vi "convert_float_array_to_U8_Picture.vi"(7 "Pict Refnum":refnum<vi>, 8 "error in (no error)":errorcluster, 9 "planeToDisplayFeatures":enum16{"XY", "XZ", "YZ"}(ring), 10 "FEATURES (PIX)":sgl[][](array[numeric]), 11 "HOLO":sgl[][](array[numeric])) -> (0 "error out":errorcluster, 3 "new picture":picture)   [LabVIEW 2023, in "holoPyTracks.lvlib"]
uses:
  holoPyTracks.lvlib
panel:
  in  "LOG?":bool=TRUE
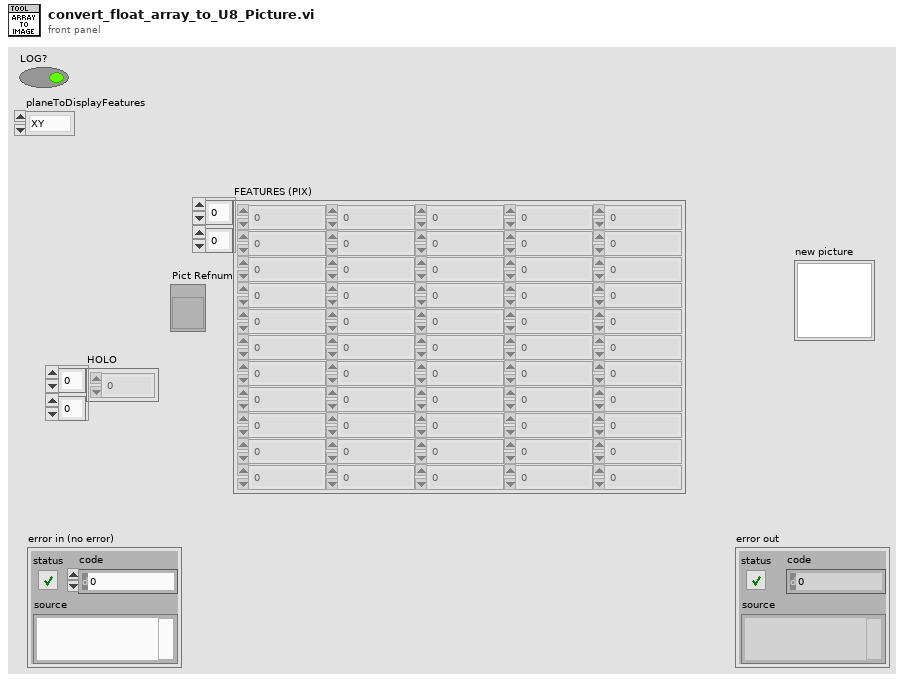
[diagram p1: front panel]
types:
  T1 = typedef "LVBoundsTypeDef.ctl" = cluster{"Width":u32, "Height":u32}
  T2 = typedef "imagedata.ctl" = cluster{"image type":i32, "image depth":i32, "image":u8[], "mask":u8[], "colors":u32[], "Rectangle":cluster{"left":i16, "top":i16, "right":i16, "bottom":i16}}
  T3 = cluster{"Width":u16, "Style":enum32{"Solid", "Dash", "Dot", "DashDot", "DashDotDot"}}
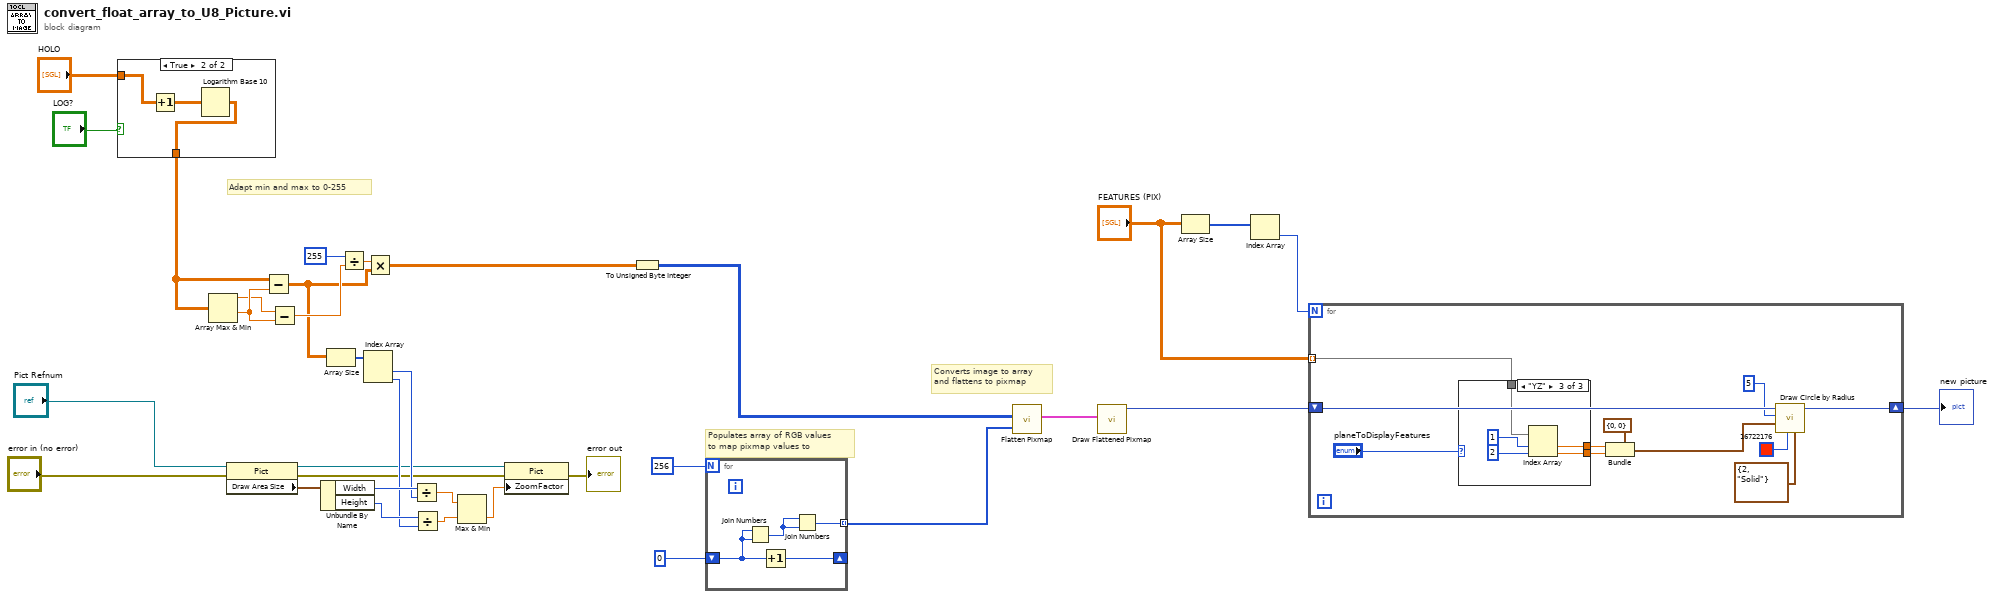
[diagram p0: block diagram]
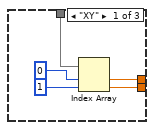
[diagram p3: hidden frame]
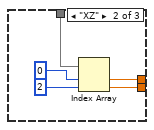
[diagram p4: hidden frame]
diagram:
  # "Adapt min and max to 0-255"
  # "Converts image to array\nand flattens to pixmap"
  # "Populates array of RGB values\nto map pixmap values to"
  n1 = case shown="True" "LOG?" {
    tunnel: "HOLO" -> [w35 w37]
    tunnel: [w35 w36] -> w2
    frame False {
    }
    frame True {
      n2 = Increment(x=w37) -> (x+1=w38:sgl[][])
      n3 = Logarithm Base 10(1:w38) -> (0:w36:sgl[][])
    }
  }
  n4 = Array Max & Min(array=w2) -> (max value=w26:sgl, min value=w27:sgl)  [unwired: 2 out]
  n5 = property on="Property Node" class="Pict"(reference="Pict Refnum", error in="error in (no error)") -> (reference out=w6:refnum<vi>, error out=w7:errorcluster, "Draw Area Size"=w24:T1)
  n6 = Subtract(x=w2, y=w27) -> (x-y=w15:sgl[][])
  n7 = Subtract(x=w26, y=w27) -> (x-y=w28:sgl)
  n8 = Unbundle By Name(w24) -> ("Width"=w23:u32, "Height"=w22:u32)
  n9 = Array Size(array=w15) -> (size(s)=w21:i32[])
  n10 = Divide(x=255, y=w28) -> (x/y=w29:sgl)
  n11 = Index Array(array=w21) -> (element #1=w20:i32, element #2=w19:i32)  [unwired: 2 in]
  n12 = Multiply(x=w29, y=w15) -> (x*y=w4:sgl[][])
  n13 = Divide(x=w23, y=w20) -> (x/y=w17:dbl)
  n14 = Divide(x=w22, y=w19) -> (x/y=w18:dbl)
  n15 = Max & Min(x=w17, y=w18) -> (min(x,y)=w16:dbl)  [unwired: 1 out]
  n16 = property on="Property Node" class="Pict"(reference=w6, error in=w7, "ZoomFactor"=w16) -> (error out=→"error out":errorcluster)  [unwired: 1 out]
  n17 = To Unsigned Byte Integer(number=w4) -> (unsigned 8bit integer=w34:u8[][])
  n18 = for {
    N: 256 -> [_]
    tunnel: [w42] -> w31 mode=indexing
    shift-right: [w41] -> _
    shift-left: u8 0 -> [w39]
    n19 = Join Numbers(hi=w39, lo=w39) -> ((hi.lo)=w40:u16)
    n20 = Increment(x=w39) -> (x+1=w41:u8)
    n21 = Join Numbers(hi=w40, lo=w40) -> ((hi.lo)=w42:u32)
  }
  n22 = call <vilib>:"Flatten Pixmap.vi"("colors"=w31, "8-bit pixmap"=w34) -> ("image data"=w30:T2)  [unwired: 9 in]
  n23 = call <vilib>:"Draw Flattened Pixmap.vi"("image data"=w30) -> ("new picture"=w14:picture)  [unwired: 8 in]
  n24 = Array Size(array="FEATURES (PIX)") -> (size(s)=w12:i32[])
  n25 = Index Array(array=w12) -> (element=w11:i32)  [unwired: 1 in]
  n26 = for {
    N: w11 -> [_]
    shift-right: [w52] -> w13
    shift-left: w14 -> [w53]
    tunnel: "FEATURES (PIX)" -> [w51] mode=indexing
    n27 = case shown="\"YZ\"" "planeToDisplayFeatures" {
      tunnel: w51 -> [w58 w63 w68]
      tunnel: [w55 w60 w65] -> w50
      tunnel: [w54 w59 w64] -> w49
      frame "XY" {
        n28 = Index Array(array=w58, index #1=0 ("disabled index (col)"), index #2=1 ("index (col)")) -> (element #1=w54:sgl, element #2=w55:sgl)
      }
      frame "XZ" {
        n29 = Index Array(array=w63, index #1=0 ("disabled index (col)"), index #2=2 ("index (col)")) -> (element #1=w59:sgl, element #2=w60:sgl)
      }
      frame "YZ" {
        n30 = Index Array(array=w68, index #1=1 ("disabled index (col)"), index #2=2 ("index (col)")) -> (element #1=w64:sgl, element #2=w65:sgl)
      }
    }
    n31 = Bundle(cluster=cluster{"horizontal":i16, "vertical":i16} {"horizontal"=0, "vertical"=0} ("pixel center"), "horizontal"=w49, "vertical"=w50) -> (w47:cluster{"horizontal":i16, "vertical":i16})
    n32 = call <vilib>:"Draw Circle by Radius.vi"("pen"=T3 {"Width"=2, "Style"=enum."Solid"}, "color(black)"=u32 16722176, "pixel center"=w47, "radius"=i16 5, "picture"=w53) -> ("new picture"=w52:picture)  [unwired: 6 in]
  }
  "new picture" <- w13
